vi "Translator.vi"(0 "Input":variant, 11 "error in (no error)":errorcluster) -> (4 "Output":variant, 15 "error out":errorcluster)   [LabVIEW 2014, in "Arduino SoftwareSerial Wrapper.lvlib"]
doc: "An example of how to create the Translator to convert the LabVIEW VIs to Arduino C code."
uses:
  Arduino SoftwareSerial Wrapper.lvlib
panel:
  out "Outputs":string[](array[string])
  out "Inputs":string[](array[string])
  out "Output Datatypes":string[](array[string])
  out "Input Datatypes":string[](array[string])
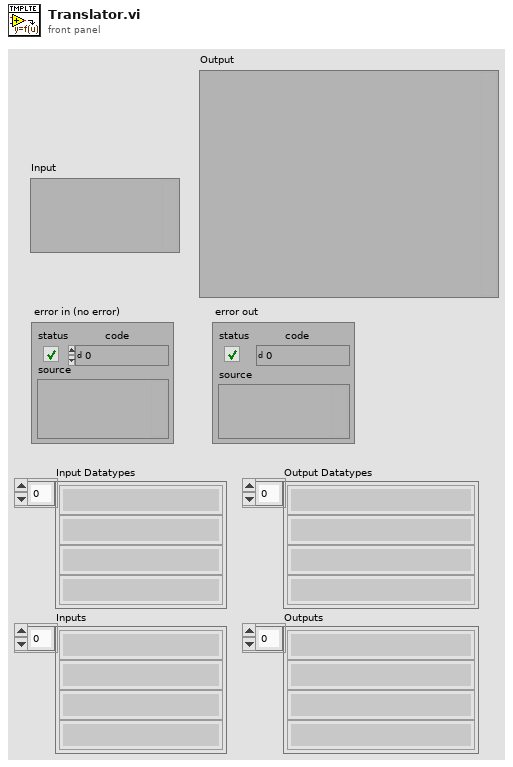
[diagram p1: front panel]
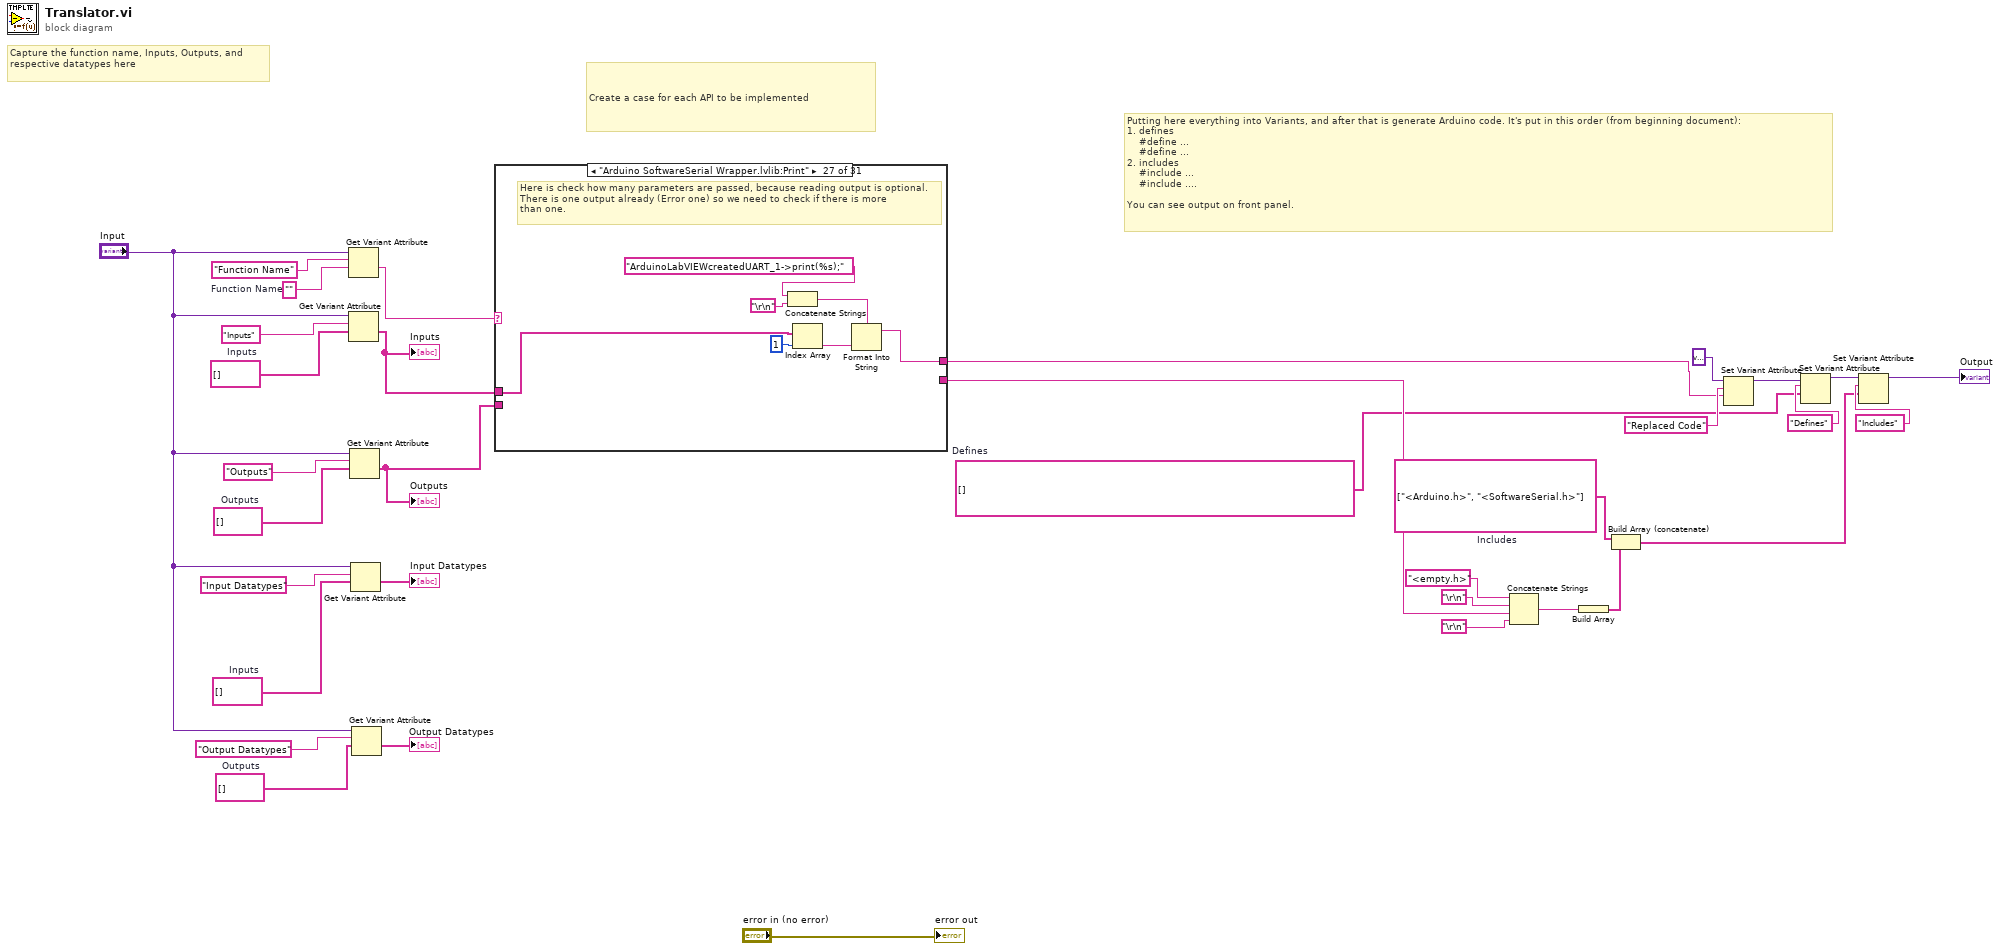
[diagram p0: block diagram]
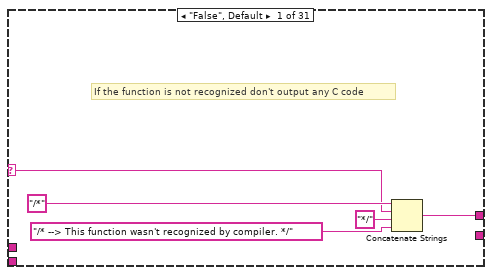
[diagram p2: hidden frame]
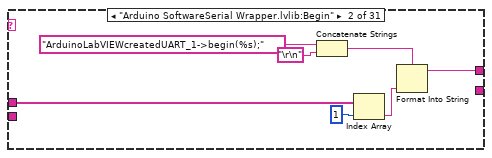
[diagram p3: hidden frame]
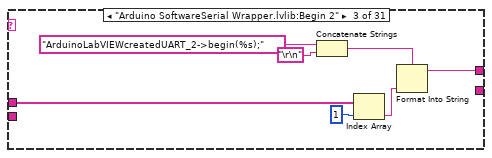
[diagram p4: hidden frame]
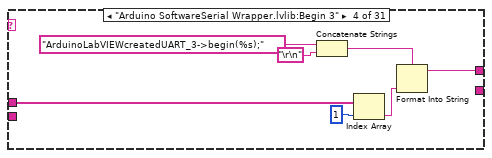
[diagram p5: hidden frame]
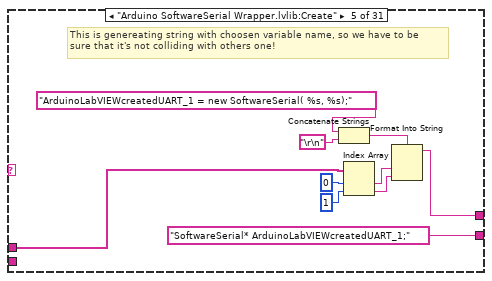
[diagram p6: hidden frame]
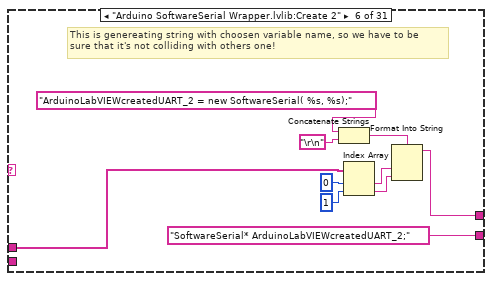
[diagram p7: hidden frame]
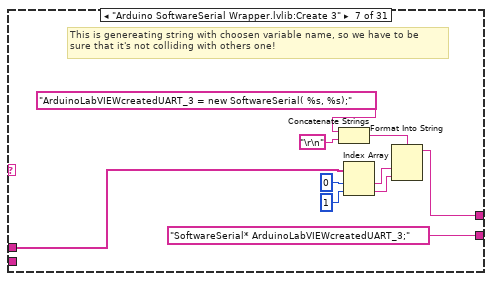
[diagram p8: hidden frame]
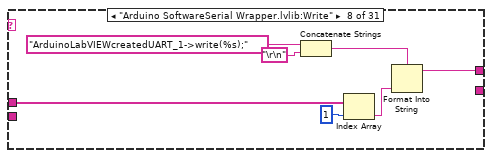
[diagram p9: hidden frame]
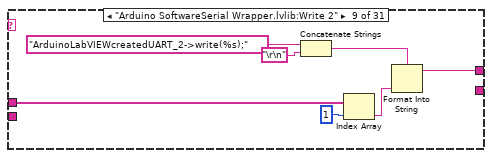
[diagram p10: hidden frame]
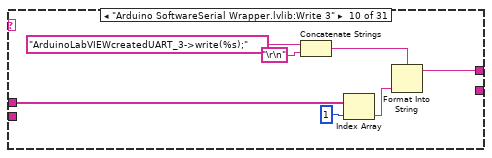
[diagram p11: hidden frame]
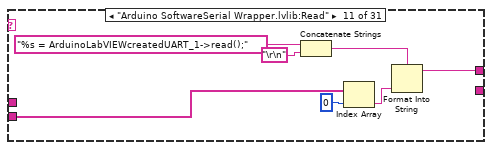
[diagram p12: hidden frame]
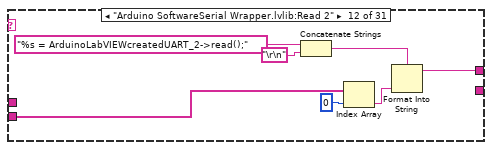
[diagram p13: hidden frame]
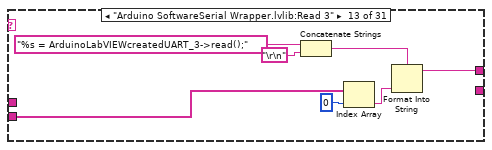
[diagram p14: hidden frame]
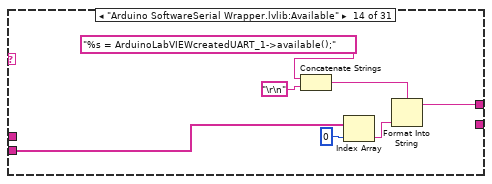
[diagram p15: hidden frame]
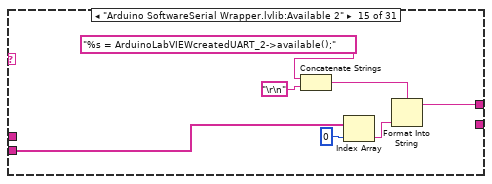
[diagram p16: hidden frame]
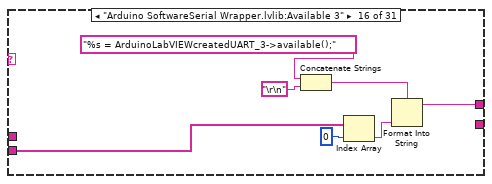
[diagram p17: hidden frame]
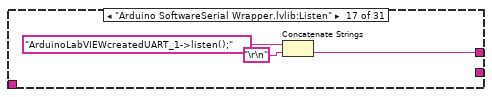
[diagram p18: hidden frame]
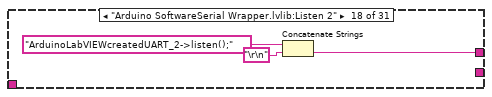
[diagram p19: hidden frame]
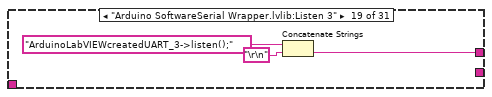
[diagram p20: hidden frame]
diagram:
  w1 = string[] []  # Defines
  w21 = string[] []  # Outputs
  w22 = string[] []  # Inputs
  w3 = string[] ["<Arduino.h>", "<SoftwareSerial.h>"]  # Includes
  w30 = string[] []  # Outputs
  w31 = string[] []  # Inputs
  w32 = ""  # Function Name
  # "Capture the function name, Inputs, Outputs, and respective datatypes here"
  # "Putting here everything into Variants, and after that is generate Arduino code. It's put in this order (from beginning document):\n1. defines\n    #define ...\n    #define ...\n2. includes\n    #include ...\n    #include ....\n\nYou can see output on front panel."
  # "Create a case for each API to be implemented"
  n1 = Get Variant Attribute(Variant="Input", name="Function Name", default value (empty Variant)=w32) -> (value=w27:string)  [unwired: 1 in, 3 out]
  n2 = Get Variant Attribute(Variant="Input", name="Inputs", default value (empty Variant)=w31) -> (value=w17:string[])  [unwired: 1 in, 3 out]
  "Inputs" <- w17
  n3 = Get Variant Attribute(Variant="Input", name="Outputs", default value (empty Variant)=w30) -> (value=w18:string[])  [unwired: 1 in, 3 out]
  "Outputs" <- w18
  n4 = Get Variant Attribute(Variant="Input", name="Input Datatypes", default value (empty Variant)=w22) -> (value=→"Input Datatypes":string[])  [unwired: 1 in, 3 out]
  n5 = Get Variant Attribute(Variant="Input", name="Output Datatypes", default value (empty Variant)=w21) -> (value=→"Output Datatypes":string[])  [unwired: 1 in, 3 out]
  n6 = case shown="\"Arduino SoftwareSerial Wrapper.lvlib:Print\"" w27 {
    selector: w27 -> [w37 _ _ _ _ _ _ _ _ _ _ _ _ _ _ _ _ _ _ _ _ _ _ _ _ _ _ _ _ _ _]
    tunnel: [w35 w46 w53 w60 w64 w74 w84 w96 w103 w110 w117 w124 w131 w139 w146 w153 w154 w157 w160 w163 w170 w177 w184 w191 w198 w214 w221 w228 w235 w245 w255] -> w26
    tunnel: w17 -> [_ w40 w47 w54 w63 w73 w83 w97 w104 w111 _ _ _ _ _ _ _ _ _ _ _ _ _ _ _ w213 w220 w227 w234 w244 w254]
    tunnel: w18 -> [_ _ _ _ _ _ _ _ _ _ w118 w125 w132 w135 w142 w149 _ _ _ w164 w171 w178 w185 w192 w199 w212 _ _ _ w243 w253]
    tunnel: [_ _ _ _ "SoftwareSerial* ArduinoLabVIEWcreatedUART_1;" "SoftwareSerial* ArduinoLabVIEWcreatedUART_2;" "SoftwareSerial* ArduinoLabVIEWcreatedUART_3;" _ _ _ _ _ _ _ _ _ _ _ _ _ _ _ _ _ _ _ _ _ _ _ _] -> w9
    frame "False", Default {
      # "If the function is not recognized don't output any C code"
      n7 = Concatenate Strings("/*" ("name"), w37, "*/" ("name"), "/* --> This function wasn't recognized by compiler. */" ("name")) -> (w35:string)
    }
    frame "Arduino SoftwareSerial Wrapper.lvlib:Begin" {
      n8 = Concatenate Strings("ArduinoLabVIEWcreatedUART_1->begin(%s);" ("name"), "\r\n") -> (w42:string)
      n9 = Index Array(array=w40, index=1) -> (element=w41:string)
      n10 = Format Into String(format string=w42, w41) -> (resulting string=w46:string)  [unwired: 2 in, 1 out]
    }
    frame "Arduino SoftwareSerial Wrapper.lvlib:Begin 2" {
      n11 = Concatenate Strings("ArduinoLabVIEWcreatedUART_2->begin(%s);" ("name"), "\r\n") -> (w49:string)
      n12 = Index Array(array=w47, index=1) -> (element=w48:string)
      n13 = Format Into String(format string=w49, w48) -> (resulting string=w53:string)  [unwired: 2 in, 1 out]
    }
    frame "Arduino SoftwareSerial Wrapper.lvlib:Begin 3" {
      n14 = Concatenate Strings("ArduinoLabVIEWcreatedUART_3->begin(%s);" ("name"), "\r\n") -> (w56:string)
      n15 = Index Array(array=w54, index=1) -> (element=w55:string)
      n16 = Format Into String(format string=w56, w55) -> (resulting string=w60:string)  [unwired: 2 in, 1 out]
    }
    frame "Arduino SoftwareSerial Wrapper.lvlib:Create" {
      # "This is genereating string with choosen variable name, so we have to be\nsure that it's not colliding with others one!"
      n17 = Concatenate Strings("ArduinoLabVIEWcreatedUART_1 = new SoftwareSerial( %s, %s);" ("name"), "\r\n") -> (w68:string)
      n18 = Index Array(array=w63, index #1=0 ("index"), index #2=1 ("index")) -> (element #1=w62:string, element #2=w65:string)
      n19 = Format Into String(format string=w68, w62, w65) -> (resulting string=w64:string)  [unwired: 2 in, 1 out]
    }
    frame "Arduino SoftwareSerial Wrapper.lvlib:Create 2" {
      # "This is genereating string with choosen variable name, so we have to be\nsure that it's not colliding with others one!"
      n20 = Concatenate Strings("ArduinoLabVIEWcreatedUART_2 = new SoftwareSerial( %s, %s);" ("name"), "\r\n") -> (w78:string)
      n21 = Index Array(array=w73, index #1=0 ("index"), index #2=1 ("index")) -> (element #1=w72:string, element #2=w75:string)
      n22 = Format Into String(format string=w78, w72, w75) -> (resulting string=w74:string)  [unwired: 2 in, 1 out]
    }
    frame "Arduino SoftwareSerial Wrapper.lvlib:Create 3" {
      # "This is genereating string with choosen variable name, so we have to be\nsure that it's not colliding with others one!"
      n23 = Concatenate Strings("ArduinoLabVIEWcreatedUART_3 = new SoftwareSerial( %s, %s);" ("name"), "\r\n") -> (w88:string)
      n24 = Index Array(array=w83, index #1=0 ("index"), index #2=1 ("index")) -> (element #1=w82:string, element #2=w85:string)
      n25 = Format Into String(format string=w88, w82, w85) -> (resulting string=w84:string)  [unwired: 2 in, 1 out]
    }
    frame "Arduino SoftwareSerial Wrapper.lvlib:Write" {
      n26 = Concatenate Strings("ArduinoLabVIEWcreatedUART_1->write(%s);" ("name"), "\r\n") -> (w92:string)
      n27 = Index Array(array=w97, index=1) -> (element=w91:string)
      n28 = Format Into String(format string=w92, w91) -> (resulting string=w96:string)  [unwired: 2 in, 1 out]
    }
    frame "Arduino SoftwareSerial Wrapper.lvlib:Write 2" {
      n29 = Concatenate Strings("ArduinoLabVIEWcreatedUART_2->write(%s);" ("name"), "\r\n") -> (w99:string)
      n30 = Index Array(array=w104, index=1) -> (element=w98:string)
      n31 = Format Into String(format string=w99, w98) -> (resulting string=w103:string)  [unwired: 2 in, 1 out]
    }
    frame "Arduino SoftwareSerial Wrapper.lvlib:Write 3" {
      n32 = Concatenate Strings("ArduinoLabVIEWcreatedUART_3->write(%s);" ("name"), "\r\n") -> (w106:string)
      n33 = Index Array(array=w111, index=1) -> (element=w105:string)
      n34 = Format Into String(format string=w106, w105) -> (resulting string=w110:string)  [unwired: 2 in, 1 out]
    }
    frame "Arduino SoftwareSerial Wrapper.lvlib:Read" {
      n35 = Concatenate Strings("%s = ArduinoLabVIEWcreatedUART_1->read();" ("name"), "\r\n") -> (w113:string)
      n36 = Index Array(array=w118, index=0) -> (element=w112:string)
      n37 = Format Into String(format string=w113, w112) -> (resulting string=w117:string)  [unwired: 2 in, 1 out]
    }
    frame "Arduino SoftwareSerial Wrapper.lvlib:Read 2" {
      n38 = Concatenate Strings("%s = ArduinoLabVIEWcreatedUART_2->read();" ("name"), "\r\n") -> (w120:string)
      n39 = Index Array(array=w125, index=0) -> (element=w119:string)
      n40 = Format Into String(format string=w120, w119) -> (resulting string=w124:string)  [unwired: 2 in, 1 out]
    }
    frame "Arduino SoftwareSerial Wrapper.lvlib:Read 3" {
      n41 = Concatenate Strings("%s = ArduinoLabVIEWcreatedUART_3->read();" ("name"), "\r\n") -> (w127:string)
      n42 = Index Array(array=w132, index=0) -> (element=w126:string)
      n43 = Format Into String(format string=w127, w126) -> (resulting string=w131:string)  [unwired: 2 in, 1 out]
    }
    frame "Arduino SoftwareSerial Wrapper.lvlib:Available" {
      n44 = Concatenate Strings("%s = ArduinoLabVIEWcreatedUART_1->available();" ("name"), "\r\n") -> (w136:string)
      n45 = Index Array(array=w135, index=0) -> (element=w134:string)
      n46 = Format Into String(format string=w136, w134) -> (resulting string=w139:string)  [unwired: 2 in, 1 out]
    }
    frame "Arduino SoftwareSerial Wrapper.lvlib:Available 2" {
      n47 = Concatenate Strings("%s = ArduinoLabVIEWcreatedUART_2->available();" ("name"), "\r\n") -> (w143:string)
      n48 = Index Array(array=w142, index=0) -> (element=w141:string)
      n49 = Format Into String(format string=w143, w141) -> (resulting string=w146:string)  [unwired: 2 in, 1 out]
    }
    frame "Arduino SoftwareSerial Wrapper.lvlib:Available 3" {
      n50 = Concatenate Strings("%s = ArduinoLabVIEWcreatedUART_3->available();" ("name"), "\r\n") -> (w150:string)
      n51 = Index Array(array=w149, index=0) -> (element=w148:string)
      n52 = Format Into String(format string=w150, w148) -> (resulting string=w153:string)  [unwired: 2 in, 1 out]
    }
    frame "Arduino SoftwareSerial Wrapper.lvlib:Listen" {
      n53 = Concatenate Strings("ArduinoLabVIEWcreatedUART_1->listen();" ("name"), "\r\n") -> (w154:string)
    }
    frame "Arduino SoftwareSerial Wrapper.lvlib:Listen 2" {
      n54 = Concatenate Strings("ArduinoLabVIEWcreatedUART_2->listen();" ("name"), "\r\n") -> (w157:string)
    }
    frame "Arduino SoftwareSerial Wrapper.lvlib:Listen 3" {
      n55 = Concatenate Strings("ArduinoLabVIEWcreatedUART_3->listen();" ("name"), "\r\n") -> (w160:string)
    }
    frame "Arduino SoftwareSerial Wrapper.lvlib:IsListening" {
      n56 = Concatenate Strings("%s = ArduinoLabVIEWcreatedUART_1->isListening();" ("name"), "\r\n") -> (w167:string)
      n57 = Index Array(array=w164, index=0) -> (element=w166:string)
      n58 = Format Into String(format string=w167, w166) -> (resulting string=w163:string)  [unwired: 2 in, 1 out]
    }
    frame "Arduino SoftwareSerial Wrapper.lvlib:IsListening 2" {
      n59 = Concatenate Strings("%s = ArduinoLabVIEWcreatedUART_2->isListening();" ("name"), "\r\n") -> (w174:string)
      n60 = Index Array(array=w171, index=0) -> (element=w173:string)
      n61 = Format Into String(format string=w174, w173) -> (resulting string=w170:string)  [unwired: 2 in, 1 out]
    }
    frame "Arduino SoftwareSerial Wrapper.lvlib:IsListening 3" {
      n62 = Concatenate Strings("%s = ArduinoLabVIEWcreatedUART_3->isListening();" ("name"), "\r\n") -> (w181:string)
      n63 = Index Array(array=w178, index=0) -> (element=w180:string)
      n64 = Format Into String(format string=w181, w180) -> (resulting string=w177:string)  [unwired: 2 in, 1 out]
    }
    frame "Arduino SoftwareSerial Wrapper.lvlib:Overflow" {
      n65 = Concatenate Strings("%s = ArduinoLabVIEWcreatedUART_1->overflow();" ("name"), "\r\n") -> (w188:string)
      n66 = Index Array(array=w185, index=0) -> (element=w189:string)
      n67 = Format Into String(format string=w188, w189) -> (resulting string=w184:string)  [unwired: 2 in, 1 out]
    }
    frame "Arduino SoftwareSerial Wrapper.lvlib:Overflow 2" {
      n68 = Concatenate Strings("%s = ArduinoLabVIEWcreatedUART_2->overflow();" ("name"), "\r\n") -> (w195:string)
      n69 = Index Array(array=w192, index=0) -> (element=w196:string)
      n70 = Format Into String(format string=w195, w196) -> (resulting string=w191:string)  [unwired: 2 in, 1 out]
    }
    frame "Arduino SoftwareSerial Wrapper.lvlib:Overflow 3" {
      n71 = Concatenate Strings("%s = ArduinoLabVIEWcreatedUART_3->overflow();" ("name"), "\r\n") -> (w202:string)
      n72 = Index Array(array=w199, index=0) -> (element=w203:string)
      n73 = Format Into String(format string=w202, w203) -> (resulting string=w198:string)  [unwired: 2 in, 1 out]
    }
    frame "Arduino SoftwareSerial Wrapper.lvlib:PrintWithReturn" {
      # "Here is check how many parameters are passed, because reading output is optional.\nThere is one output already (Error one) so we need to check if there is more\nthan one."
      n74 = Concatenate Strings("%s = ArduinoLabVIEWcreatedUART_1->print(%s);" ("name"), "\r\n") -> (w210:string)
      n75 = Index Array(array=w213, index=1) -> (element=w205:string)
      n76 = Index Array(array=w212, index=0) -> (element=w206:string)
      n77 = Format Into String(format string=w210, w206, w205) -> (resulting string=w214:string)  [unwired: 2 in, 1 out]
    }
    frame "Arduino SoftwareSerial Wrapper.lvlib:Print" {
      # "Here is check how many parameters are passed, because reading output is optional.\nThere is one output already (Error one) so we need to check if there is more\nthan one."
      n78 = Concatenate Strings("ArduinoLabVIEWcreatedUART_1->print(%s);" ("name"), "\r\n") -> (w218:string)
      n79 = Index Array(array=w220, index=1) -> (element=w215:string)
      n80 = Format Into String(format string=w218, w215) -> (resulting string=w221:string)  [unwired: 2 in, 1 out]
    }
    frame "Arduino SoftwareSerial Wrapper.lvlib:Print 2" {
      # "Here is check how many parameters are passed, because reading output is optional.\nThere is one output already (Error one) so we need to check if there is more\nthan one."
      n81 = Concatenate Strings("ArduinoLabVIEWcreatedUART_2->print(%s);" ("name"), "\r\n") -> (w225:string)
      n82 = Index Array(array=w227, index=1) -> (element=w222:string)
      n83 = Format Into String(format string=w225, w222) -> (resulting string=w228:string)  [unwired: 2 in, 1 out]
    }
    frame "Arduino SoftwareSerial Wrapper.lvlib:Print 3" {
      # "Here is check how many parameters are passed, because reading output is optional.\nThere is one output already (Error one) so we need to check if there is more\nthan one."
      n84 = Concatenate Strings("ArduinoLabVIEWcreatedUART_3->print(%s);" ("name"), "\r\n") -> (w232:string)
      n85 = Index Array(array=w234, index=1) -> (element=w229:string)
      n86 = Format Into String(format string=w232, w229) -> (resulting string=w235:string)  [unwired: 2 in, 1 out]
    }
    frame "Arduino SoftwareSerial Wrapper.lvlib:PrintWithReturn 2" {
      # "Here is check how many parameters are passed, because reading output is optional.\nThere is one output already (Error one) so we need to check if there is more\nthan one."
      n87 = Concatenate Strings("%s = ArduinoLabVIEWcreatedUART_2->print(%s);" ("name"), "\r\n") -> (w241:string)
      n88 = Index Array(array=w244, index=1) -> (element=w236:string)
      n89 = Index Array(array=w243, index=0) -> (element=w237:string)
      n90 = Format Into String(format string=w241, w237, w236) -> (resulting string=w245:string)  [unwired: 2 in, 1 out]
    }
    frame "Arduino SoftwareSerial Wrapper.lvlib:PrintWithReturn 3" {
      # "Here is check how many parameters are passed, because reading output is optional.\nThere is one output already (Error one) so we need to check if there is more\nthan one."
      n91 = Concatenate Strings("%s = ArduinoLabVIEWcreatedUART_3->print(%s);" ("name"), "\r\n") -> (w251:string)
      n92 = Index Array(array=w254, index=1) -> (element=w246:string)
      n93 = Index Array(array=w253, index=0) -> (element=w247:string)
      n94 = Format Into String(format string=w251, w247, w246) -> (resulting string=w255:string)  [unwired: 2 in, 1 out]
    }
  }
  n95 = Concatenate Strings("<empty.h>" ("string"), "\r\n", w9, "\r\n") -> (w12:string)
  n96 = Build Array(w12) -> (w2:string[])
  n97 = Build Array (concatenate)(w3, w2) -> (w4:string[])
  n98 = Set Variant Attribute(Variant=variant ("variant"), name="Replaced Code", value=w26) -> (Variant out=w7:variant)  [unwired: 1 in, 2 out]
  n99 = Set Variant Attribute(Variant=w7, name="Defines", value=w1) -> (Variant out=w6:variant)  [unwired: 1 in, 2 out]
  n100 = Set Variant Attribute(Variant=w6, name="Includes", value=w4) -> (Variant out=→"Output":variant)  [unwired: 1 in, 2 out]
  "error out" <- "error in (no error)"
